vi "GPS Read (Poly).vi"   [LabVIEW 2009]
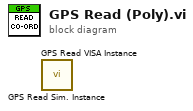
[diagram p0: block diagram]
diagram:
  n1 = call "GPS Read Sim. Instance.vi"() -> ()  [unwired: 13 in, 7 out]
  n2 = call "GPS Read VISA Instance.vi"() -> ()  [unwired: 13 in, 7 out]
